vi "Sub VI Straight PID Gyro.vi"(10 "NXT/EV3":T1, 11 "PortGyro":T2 items=["Port 1", "Port 2", "Port 3", "Port 4"]) -> (2 "NXT/EV3 2":T1)   [LabVIEW 2016]
uses:
  <vilib>/NXT/Subs/LVHSConnector.ctl
  <vilib>/NXT/LegoClasses/BrickReference/BrickReference.lvclass
  <vilib>/NXT/Block Support/NXT_InputPort.ctl
  <vilib>/NXT/Block Support/NXT_ButtonSelector.ctl
  <vilib>/NXT/Block Support/NXT_OutputPort.ctl
  <vilib>/NXT/Dual Mode Library/Sensors/EV3_Gyro_Angle.vi
  <vilib>/NXT/NXTIO Xnodes/NXTIONodeSubVIs/NXTMoveMotors.vi
  <vilib>/NXT/Dual Mode Library/Sensors/readNXTButton.vi
  <vilib>/NXT/NXTIO Xnodes/AddressXNode/NXTIOAddress.xnode
  <vilib>/NXT/NXTIO Xnodes/NXTIOXNode/NXTIO.xnode
panel:
  in  "inicial":sgl
  in  "Kd":sgl
  in  "Ki":sgl
  in  "Kp":sgl=2.0
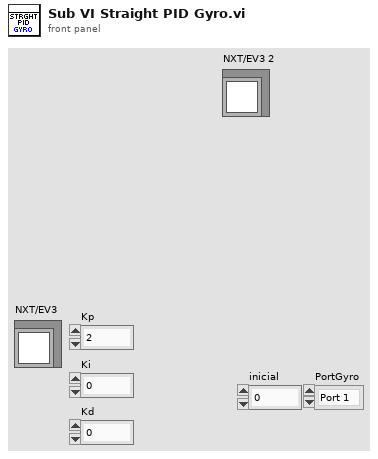
[diagram p1: front panel]
types:
  T1 = typedef "LVHSConnector.ctl" = refnum<class "BrickReference.lvclass">
  T2 = typedef "NXT_InputPort.ctl" = u32
  T3 = typedef "NXT_OutputPort.ctl" = u8
  T4 = typedef "NXT_ButtonSelector.ctl" = u16
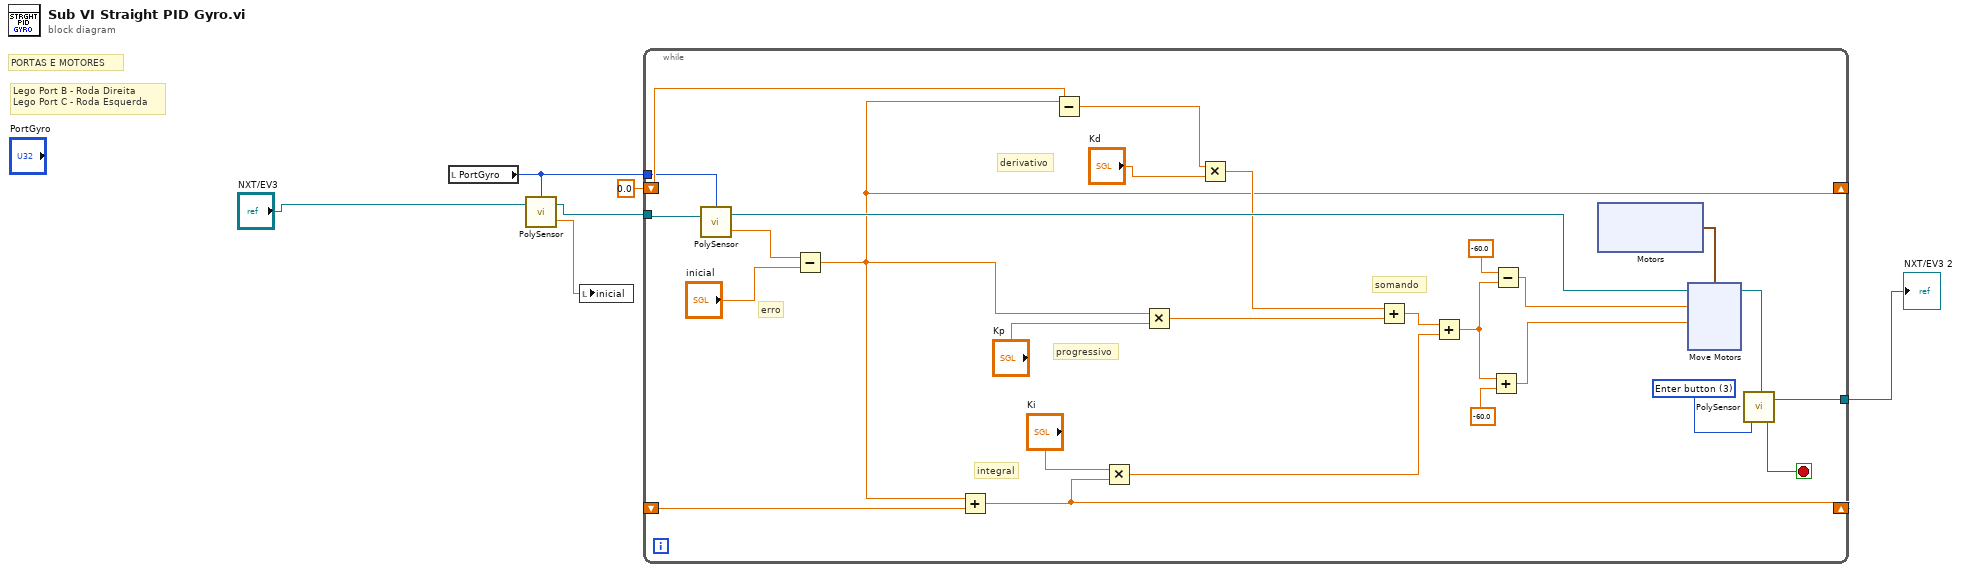
[diagram p0: block diagram]
diagram:
  # "Lego Port B - Roda Direita\nLego Port C - Roda Esquerda"
  # "PORTAS E MOTORES"
  n1 = local read "PortGyro"() -> (w3:T2)
  n2 = call-poly <vilib>:"PolySensor.vi"("NXT/EV3"="NXT/EV3", "Port (Port 1)"=w3) -> ("Degrees"=w5:sgl, "NXT/EV3"=w6:T1)  [unwired: 1 in]
  n3 = local write "inicial"(w5) -> ()
  n4 = while {
    tunnel: w6 -> [w33]
    shift-right: [w17] -> _
    shift-left: _ -> [w19]
    shift-right: [w11] -> _
    shift-left: sgl 0.0 -> [w14]
    tunnel: w3 -> [w8]
    tunnel: [w7] -> w1
    stop <- w31 stop-if-true
    w32 = T4 3 items=["Enter button"=3, "Left button"=2, "Right button"=1] ("Button (Enter button)")
    # "somando"
    # "erro"
    # "progressivo"
    # "integral"
    # "derivativo"
    n5 = call-poly <vilib>:"PolySensor.vi"("NXT/EV3"=w33, "Port (Port 1)"=w8) -> ("Degrees"=w13:sgl, "NXT/EV3"=w21:T1)  [unwired: 1 in]
    n6 = Subtract(x=w13, y="inicial") -> (x-y=w11:sgl)
    n7 = Add(x=w11, y=w19) -> (x+y=w17:sgl)
    n8 = Subtract(x=w11, y=w14) -> (x-y=w9:sgl)
    n9 = Multiply(x="Ki", y=w17) -> (x*y=w16:sgl)
    n10 = Multiply(x=w11, y="Kp") -> (x*y=w24:sgl)
    n11 = Multiply(x=w9, y="Kd") -> (x*y=w15:sgl)
    n12 = Add(x=w15, y=w24) -> (x+y=w22:sgl)
    n13 = Add(x=w22, y=w16) -> (x+y=w23:sgl)
    n14 = Add(x=w23, y=sgl -60.0) -> (x+y=w25:sgl)
    n15 = Subtract(x=sgl -60.0, y=w23) -> (x-y=w28:sgl)
    n16 = xnode "Motors"() -> ("Motor"=w30:cluster{"Port":T3, "Port":T3})
    n17 = xnode "Move Motors"("Power/Speed 2"=w25, "Power/Speed 1"=w28, "Motors"=w30, "NXT/EV3"=w21) -> ("NXT/EV3"=w20:T1)
    n18 = call-poly <vilib>:"PolySensor.vi"("Button (Enter button)"=w32, "NXT/EV3"=w20) -> ("Yes/No"=w31:bool, "NXT/EV3"=w7:T1)  [unwired: 1 out]
  }
  "NXT/EV3 2" <- w1
